vi "Get_Audio_Devices.vi"(4 "error in":errorcluster, 5 "OptionalAttributes":string, 6 "RequiredAttributes":string, 7 "SpeechLib.ISpeechVoice (In)":refnum<k7>) -> (0 "error out":errorcluster, 1 "AudioDevices":string[](array[string]), 2 "GetAudioOutputs":refnum<k7>, 3 "SpeechLib.ISpeechVoice (Out)":refnum<k7>)   [LabVIEW 8.6]
doc: "This SubVI calls the Microsoft Speech SDK 5.1 software and loads the audio devices available on your computer into an output array for use by the LVTTS.vi"
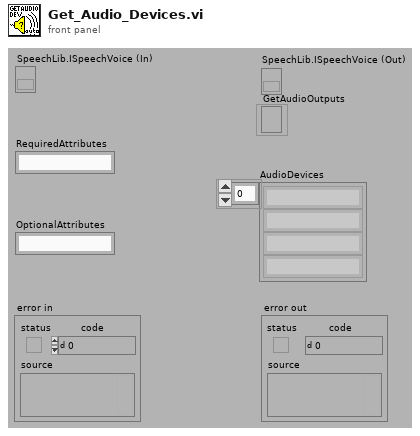
[diagram p1: front panel]
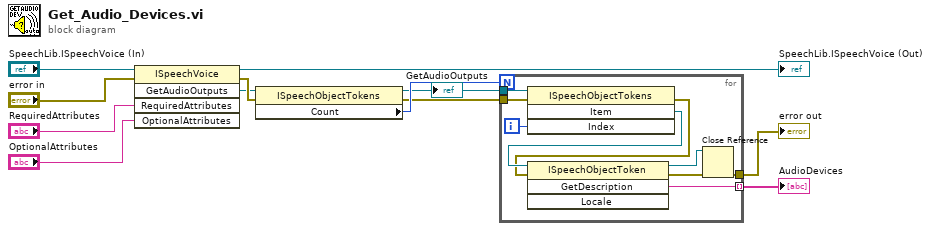
[diagram p0: block diagram]
diagram:
  n1 = invoke class="ISpeechVoice" method="GetAudioOutputs"(reference="SpeechLib.ISpeechVoice (In)", error in="error in", "RequiredAttributes"="RequiredAttributes", "OptionalAttributes"="OptionalAttributes") -> (reference out=→"SpeechLib.ISpeechVoice (Out)":refnum<k7>, error out=w5:errorcluster, "GetAudioOutputs"=w3:refnum<k7>)  [unwired: 1 in, 2 out]
  n2 = property class="ISpeechObjectTokens"(reference=w3, error in=w5) -> (reference out=w4:refnum<k7>, error out=w6:errorcluster, "Count"=w9:i32)
  "GetAudioOutputs" <- w4
  n3 = for {
    N: w9 -> [_]
    tunnel: [w13] -> w8
    tunnel: w6 -> [w18]
    tunnel: w4 -> [w17]
    tunnel: [w16] -> w7 mode=indexing
    i -> [w20]
    n4 = invoke class="ISpeechObjectTokens" method="Item"(reference=w17, error in=w18, "Index"=w20) -> (error out=w15:errorcluster, "Item"=w21:refnum<k7>)  [unwired: 1 in, 2 out]
    n5 = invoke class="ISpeechObjectToken" method="GetDescription"(reference=w21, error in=w15) -> (reference out=w19:refnum<k7>, error out=w14:errorcluster, "GetDescription"=w16:string)  [unwired: 2 in, 1 out]
    n6 = Close Reference(reference=w19, error in (no error)=w14) -> (error out=w13:errorcluster)
  }
  "error out" <- w8
  "AudioDevices" <- w7
